vi "CreateVI.vi"(0 "__args":cluster{"targetVi":string}) -> (1 "__return":i32, 2 "__errStatus":bool, 3 "__errCode":i32, 4 "__errSource":string)   [LabVIEW 2013]
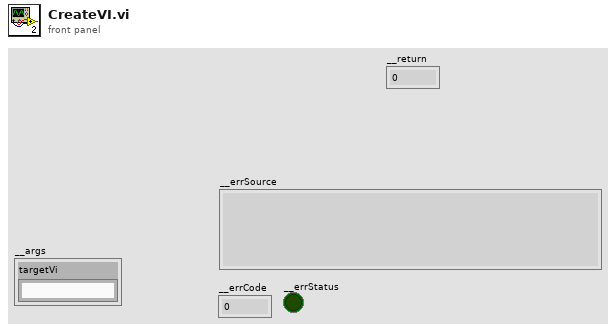
[diagram p1: front panel]
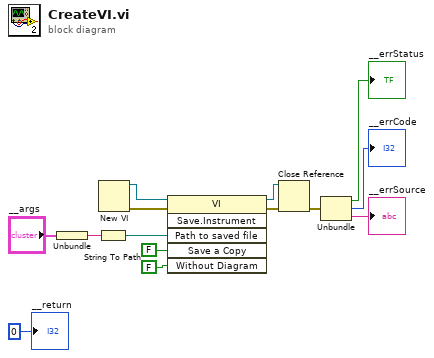
[diagram p0: block diagram]
diagram:
  n1 = Unbundle("__args") -> ("targetVi"=w2:string)
  n2 = String To Path(string=w2) -> (path=w3:path)
  n3 = New VI() -> (0:w8:errorcluster, 3:w10:refnum<vi>)  [unwired: 7 in]
  n4 = invoke class="VI" method="Save.Instrument"(reference=w10, error in=w8, "Path to saved file"=w3, "Save a Copy"=FALSE, "Without Diagram"=FALSE) -> (reference out=w9:refnum<vi>, error out=w7:errorcluster)  [unwired: 1 in, 4 out]
  n5 = Close Reference(reference=w9, error in (no error)=w7) -> (error out=w4:errorcluster)
  n6 = Unbundle(w4) -> ("status"=→"__errStatus":bool, "code"=→"__errCode":i32, "source"=→"__errSource":string)
  "__return" <- 0
